vi "Globals.vi"() -> ()   [LabVIEW 2010]
panel:
  in  "stop":bool
  out "Page Names":string[](array[string])=["First", "Second", "Third", "Fourth"]
  in  "Page":i16
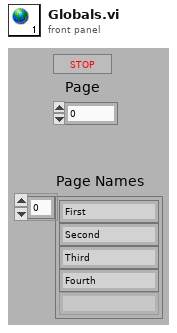
[diagram p1: front panel]
diagram:
